vi "dfd_Disable First Time Running Warning.vi"(0 "error in":errorcluster, 1 "disable?":bool=TRUE) -> (2 "error out":errorcluster)   [LabVIEW 2017, in "NI_DigFilterLicensed.lvlib"]
uses:
  <vilib>/addons/Digital Filter Design/NI_DigFilterLicensed.lvlib
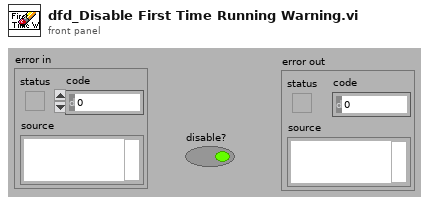
[diagram p1: front panel]
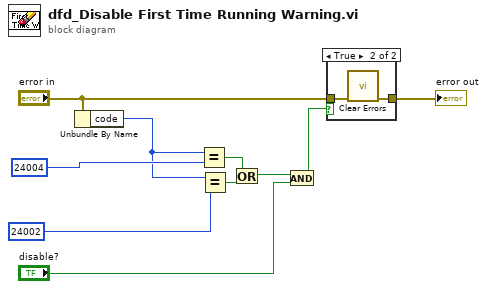
[diagram p0: block diagram]
diagram:
  n1 = Unbundle By Name("error in") -> ("code"=w3:i32)
  n2 = Equal?(x=w3, y=24004 ("WRN_STATE_EMPTY")) -> (x = y?=w4:bool)
  n3 = Equal?(x=w3, y=24002 ("WRN_TIME_STAMP_INCONSISTENT")) -> (x = y?=w1:bool)
  n4 = Or(x=w4, y=w1) -> (x .or. y?=w5:bool)
  n5 = And(x=w5, y="disable?") -> (x .and. y?=w6:bool)
  n6 = case shown="True" w6 {
    tunnel: "error in" -> [w11 w13]
    tunnel: [w11 w12] -> w9
    frame False {
    }
    frame True {
      n7 = call <vilib>:"Clear Errors.vi"("error in (no error)"=w13) -> ("error out"=w12:errorcluster)  [unwired: 1 in, 5 out]
    }
  }
  "error out" <- w9
